vi "Read VI.vi"(8 "error in (no error)":errorcluster, 11 "VI Path in":path) -> (0 "error out":errorcluster, 3 "Content out":T1)   [LabVIEW 2018, in "VI-Hacker.lvlib"]
uses:
  VI-Hacker.lvlib
  <vilib>/Utility/error.llb/Error Cluster From Error Code.vi
  <vilib>/ErrorRing/Error Ring.xnode
  TypeDefs/Block.ctl
  TypeDefs/Content.ctl
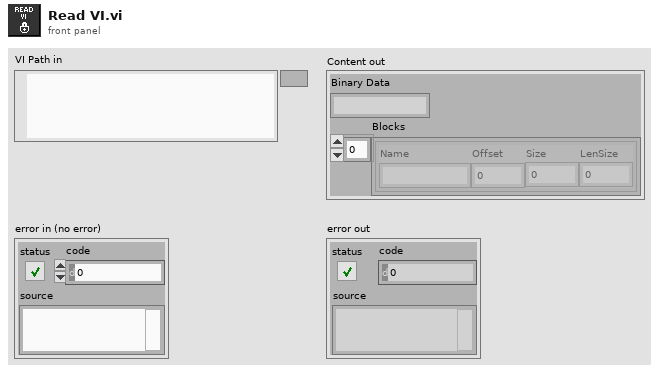
[diagram p1: front panel]
types:
  T1 = typedef "VI-Hacker.lvlib/Content.ctl" = cluster{"Binary Data":string, "Blocks":T2[]}
  T2 = typedef "VI-Hacker.lvlib/Block.ctl" = cluster{"Name":string, "Offset":i32, "Size":i32, "LenSize":i32}
  T3 = enum16{"open", "replace", "create", "open or create", "replace or create", "replace or create with confirmation"}
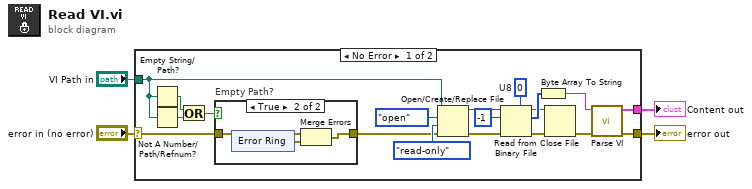
[diagram p0: block diagram]
diagram:
  n1 = case shown="No Error" "error in (no error)" {
    selector: "error in (no error)" -> [w11 w32]
    tunnel: "VI Path in" -> [w9 _]
    tunnel: [w7 w32] -> w2
    tunnel: [w5 _] -> w1
    frame No Error {
      w20 = u8 0  # U8
      n2 = Empty String/Path?(string/path=w9) -> (empty?=w13:bool)
      n3 = Not A Number/Path/Refnum?(number/path/refnum=w9) -> (NaN/Path/Refnum?=w14:bool)
      n4 = Or(x=w13, y=w14) -> (x .or. y?=w12:bool)
      n5 = case "Empty Path?" shown="True" w12 {
        tunnel: w11 -> [w24 w27]
        tunnel: [w24 w26] -> w10
        frame False {
        }
        frame True {
          n6 = xnode "Error Ring"() -> ("error out"=w25:errorcluster)
          n7 = Merge Errors(w27, w25) -> (w26:errorcluster)
        }
      }
      n8 = Open/Create/Replace File(file path (use dialog)=w9, error in=w10, operation (0:open)=T3."open", access (0:read/write)=enum16{"read/write", "read-only", "write-only"}."read-only") -> (refnum out=w15:refnum<file>, error out=w21:errorcluster)  [unwired: 3 out]
      n9 = Read from Binary File(5:w20, 8:w21, 10:-1 ("count (1)"), 11:w15) -> (0:w17:errorcluster, 2:w19:u8[], 3:w18:refnum<file>)  [unwired: 1 in, 2 out]
      n10 = Byte Array To String(unsigned byte array=w19) -> (string=w6:string)
      n11 = Close File(refnum=w18, error in=w17) -> (error out=w8:errorcluster)  [unwired: 1 out]
      n12 = call "Parse VI.vi"("error in (no error)"=w8, "VI Binary Data in"=w6) -> ("error out"=w7:errorcluster, "Content out"=w5:T1)  [unwired: 8 in]
    }
    frame Error {
    }
  }
  "error out" <- w2
  "Content out" <- w1
